vi "Set All Properties.vi"(8 "error in (no error)":errorcluster, 10 "Properties":variant, 11 "RS-xxx in":refnum<class "RS-xxx.lvclass">) -> (0 "error out":errorcluster, 3 "RS-xxx out":refnum<class "RS-xxx.lvclass">)   [LabVIEW 2019, in "Protocols.lvlib" / "RS-xxx.lvclass"]
uses:
  RS-xxx.lvclass
  Protocol Parent/Protocol Parent.lvclass
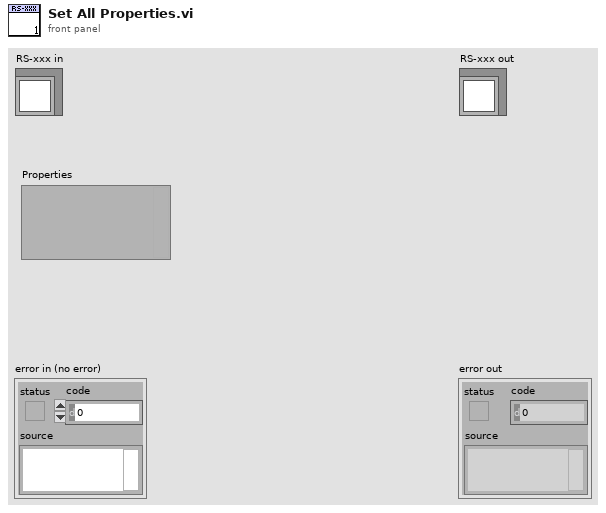
[diagram p1: front panel]
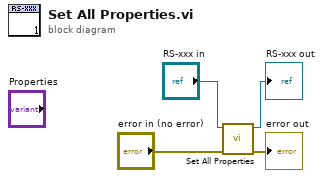
[diagram p0: block diagram]
diagram:
  n1 = call-parent "Set All Properties.vi"("error in (no error)"="error in (no error)", "Protocol Parent in"="RS-xxx in") -> ("error out"=→"error out":errorcluster, "Protocol Parent out"=→"RS-xxx out":refnum<class "RS-xxx.lvclass">)  [unwired: 8 in]
